vi "ATMonochromator_getEvent_rejectedCommand.vi"(8 "error in (no error)":errorcluster, 11 "logevent_rejectedCommand_Ctl":T1) -> (0 "error out":errorcluster, 2 "function return":i32, 3 "logevent_rejectedCommand_Ctl out":T1)   [LabVIEW 2016, in "SALLV_ATMonochromator.lvlib"]
doc: "int ATMonochromator_shm_getEvent_rejectedCommandLV(ATMonochromator_logevent_rejectedCommandLV *logevent_rejectedCommand_Ctl );"
uses:
  SALLV_ATMonochromator.lvlib
  DataTypes/logevent_rejectedCommand.ctl
  SALLV_ATMonochromator.so
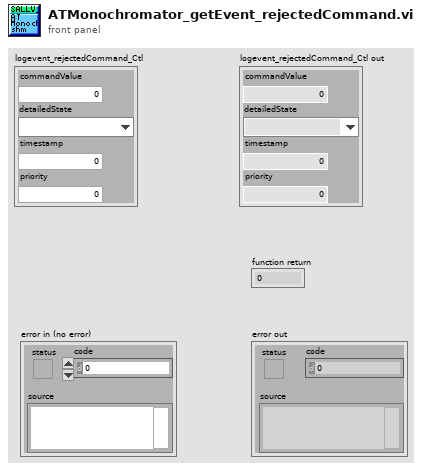
[diagram p1: front panel]
types:
  T1 = typedef "SALLV_ATMonochromator.lvlib/logevent_rejectedCommand.ctl" = cluster{"commandValue":u16, "detailedState":enum32{"", "DisabledState", "EnabledState", "FaultState", "OfflineState", "StandbyState", "MonoSettingUpState", "StoppedState", "StoppedCoolerOffState", "StoppedLightOffState", "StoppedLightOnState", "MonoManualSetup", "MonoAutomaticSetup"}, "timestamp":dbl, "priority":i32}
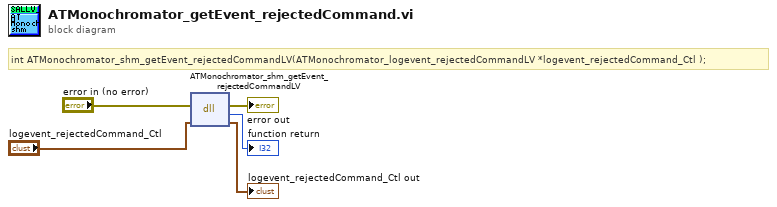
[diagram p0: block diagram]
diagram:
  # "int ATMonochromator_shm_getEvent_rejectedCommandLV(ATMonochromator_logevent_rejectedCommandLV *logevent_rejectedCommand_Ctl );"
  n1 = dll-call lib="home/harini/tcs/SALLV_ATMonochromator/SALLV_ATMonochromator.*" fn="ATMonochromator_shm_getEvent_rejectedCommandLV"(error in="error in (no error)", "logevent_rejectedCommand_Ctl"="logevent_rejectedCommand_Ctl") -> (error out=→"error out":errorcluster, →"function return":i32, "logevent_rejectedCommand_Ctl"=→"logevent_rejectedCommand_Ctl out":T1)  [unwired: 2 in, 1 out]
